vi "Done Global Log.vi"(8 "error in (no error)":errorcluster) -> (0 "error out":errorcluster)   [LabVIEW 2016, in "Stream Log.lvlib" / "Global Application Log.lvclass"]
doc: "--\nCopyright © 2017 Composed SystemsI All rights reserved.\n\nAuthor: Jon McBee <jon.mcbee@composed.io>\n\nThis library is provided \"AS IS\" ,WITHOUT WARRANTIES OR\nCONDITIONS OF ANY KIND, either express or implied.\n\nComposed Systems -- composed.io\n\nStream 0.0.1.1\nJon McBee - Composed Systems\nCopyright (c) 2017, Composed Systems"
uses:
  <userlib>/Composed Systems/Stream/Log/Global Application Log/Global Application Log.lvclass
  <userlib>/Composed Systems/Stream/Log/Global Application Log/Log Reference Action.ctl
  <userlib>/Composed Systems/Stream/Log/Global Application Log/Global Application Log.lvclass/Global Application Log.ctl
  <userlib>/Composed Systems/Stream/Log/Application Log/Application Log.lvclass
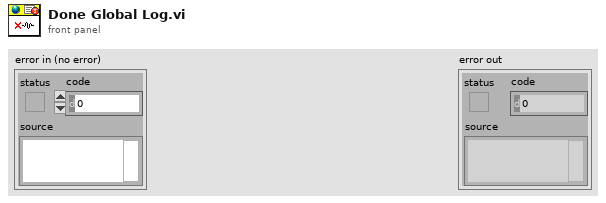
[diagram p1: front panel]
types:
  T1 = typedef "Stream Log.lvlib/Global Application Log.lvclass/Log Reference Action.ctl" = enum16{"Get Log Reference", "Set Log Reference"}
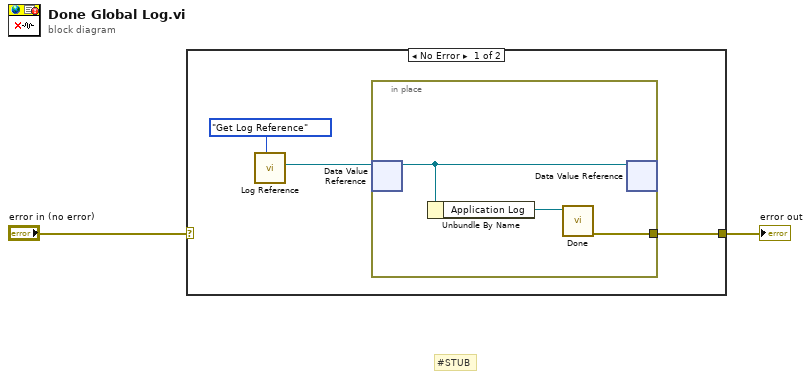
[diagram p0: block diagram]
diagram:
  # "#STUB"
  n1 = case shown="No Error" "error in (no error)" {
    selector: "error in (no error)" -> [_ w9]
    tunnel: [w3 w9] -> w1
    frame No Error {
      n2 = call <userlib>:"Log Reference.vi"("Action"=Log_Reference_Action."Get Log Reference") -> ("Global Log Reference out"=w4:refnum<data-value>)  [unwired: 10 in]
      n3 = in-place {
        in-place-border: [w6] -> w3
        n4 = in-place-dvr #1(w4) -> (w7:refnum<class "Global Application Log.lvclass">)  [unwired: 1 out]
        n5 = Unbundle By Name(w7) -> ("Application Log"=w8:refnum<class "Application Log.lvclass">)
        n6 = call-dynamic "Done.vi"("Application Log in"=w8) -> ("error out"=w6:errorcluster)  [unwired: 9 in, 1 out]
        n7 = in-place-dvr #1(w7) -> ()  [unwired: 2 out]
      }
    }
    frame Error {
    }
  }
  "error out" <- w1
